vi "mqttCmdPublishAckCommand.vi"(0 "queue":refnum<queue>, 9 "messageID":u16, 11 "error in (no error)":errorcluster) -> (15 "error out":errorcluster)   [LabVIEW 2014, in "labview-mqtt.lvlib" / "mqttCmdPublish.lvclass"]
uses:
  mqttCmdPublish.lvclass
  mqttTypedef/mqttMessageType.ctl
  mqttTypedef/mqttQOSlevel.ctl
  mqttCmd.lvclass
  labview-mqtt.lvlib
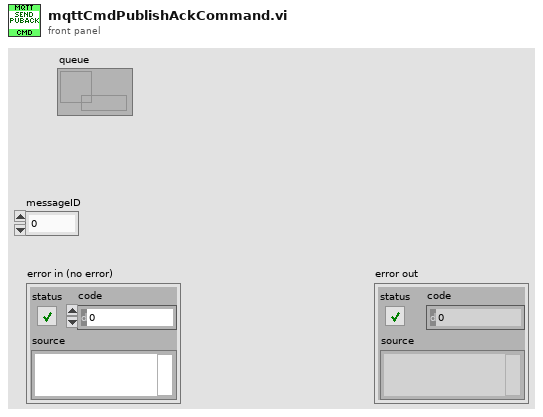
[diagram p1: front panel]
types:
  T1 = typedef "labview-mqtt.lvlib/mqttQOSlevel.ctl" = enum8{"At most once", "At least once", "Exactly once", "Reserved"}
  T2 = typedef "labview-mqtt.lvlib/mqttMessageType.ctl" = enum32{"Reserved", "CONNECT", "CONNACK", "PUBLISH", "PUBACK", "PUBREC", "PUBREL", "PUBCOMP", "SUBSCRIBE", "SUBACK", "UNSUBSCRIBE", "UNSUBACK", "PINGREQ", "PINGRESP", "DISCONNECT", "Reserved2"}
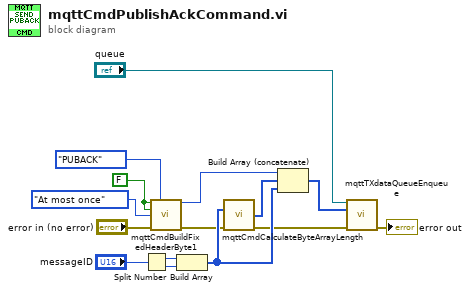
[diagram p0: block diagram]
diagram:
  w2 = FALSE ("retain(F)")
  n1 = Split Number(x="messageID") -> (hi(x)=w8:u8, lo(x)=w9:u8)
  n2 = call "mqttCmdBuildFixedHeaderByte1.vi"("retain(F)"=w2, "MessageType"=mqttMessageType."PUBACK", "duplicate(F)"=w2, "QoS (At most once)"=mqttQOSlevel."At most once", "error in (no error)"="error in (no error)") -> ("byte1"=w10:u8, "error out"=w5:errorcluster)  [unwired: 9 in]
  n3 = Build Array(w8, w9) -> (w6:u8[])
  n4 = call "mqttCmdCalculateByteArrayLength.vi"("byteArry in"=w6, "error in (no error)"=w5) -> ("length out"=w3:u8[], "error out"=w4:errorcluster)  [unwired: 12 in]
  n5 = Build Array (concatenate)(w10, w3, w6) -> (w11:u8[])
  n6 = call "mqttTXdataQueueEnqueue.vi"("queue"="queue", "data in"=w11, "error in (no error)"=w4) -> ("error out"=→"error out":errorcluster)  [unwired: 12 in]
